vi "PostSub Steps HV PPS.vi"(0 "Sequence Context In":refnum<k7>, 1 "PPS Config In":T1={"VISA Resource"="", "Voltage Level (0.0 V)"=0.0, "CURRent Limit (0.0 A)"=0.0, "OVP LEVEL (0V)"=0.0, "Enable OVP (T: Enable)"=TRUE, "OCP LEVEL (0A)"=0.0, "Enable OCP (T: Enable)"=TRUE, "Value Out"="", "Value In"="", "Actual Voltage Level (V)"=0.0, "Actual Current Limit (A)"=0.0, "Select Instrument"="", "Enable Output"=FALSE, "PPS Operation"=enum."Close", "Type"=0} {"Type" items=["Voltage", "Current"]; "Actual Current Limit (A)" format="%.2f"; "Actual Voltage Level (V)" format="%.2f"; "OCP LEVEL (0A)" format="%.2f"; "OVP LEVEL (0V)" format="%.2f"; "Voltage Level (0.0 V)" format="%.2f"}, 2 "Socket Index":i16) -> (7 "Report Text":string, 8 "PPS Config Out":T1={"VISA Resource"="", "Voltage Level (0.0 V)"=0.0, "CURRent Limit (0.0 A)"=0.0, "OVP LEVEL (0V)"=0.0, "Enable OVP (T: Enable)"=TRUE, "OCP LEVEL (0A)"=0.0, "Enable OCP (T: Enable)"=TRUE, "Value Out"="", "Value In"="", "Actual Voltage Level (V)"=0.0, "Actual Current Limit (A)"=0.0, "Select Instrument"="", "Enable Output"=FALSE, "PPS Operation"=enum."Close", "Type"=0} {"Type" items=["Voltage", "Current"]; "Actual Current Limit (A)" format="%.2f"; "Actual Voltage Level (V)" format="%.2f"; "OCP LEVEL (0A)" format="%.2f"; "OVP LEVEL (0V)" format="%.2f"; "Voltage Level (0.0 V)" format="%.2f"}, 10 "error out":errorcluster)   [LabVIEW 2023, in "LTT_TeststandSteptypes.lvlib"]
uses:
  LTT_TeststandSteptypes.lvlib
  HardwareAbstractionLayer_LVOOP/PowerSupply/Teststand/Control/PPS StepType Control.ctl
  HardwareAbstractionLayer_LVOOP/PowerSupply/Control/PPS FGV Option.ctl
  HardwareAbstractionLayer_LVOOP/PowerSupply/Control/PPS Configure Data.ctl
  HardwareAbstractionLayer_LVOOP/PowerSupply/IT-M6018C/IT-M6018C.lvclass
  D:/eDCU LTT/VT LTT Project/Source Code/HardwareAbstractionLayer_LVOOP/PowerSupply/PowerSupply.lvclass
  <vilib>/addons/TestStand/_TSUtility.llb/TestStand - Set Property Value (Number).vi
  HardwareAbstractionLayer_LVOOP/PowerSupply/PowerSupply.lvclass
  HardwareAbstractionLayer_LVOOP/PowerSupply/IT-M3904D/IT-M3904D.lvclass
  HardwareAbstractionLayer_LVOOP/Database/Database.lvclass
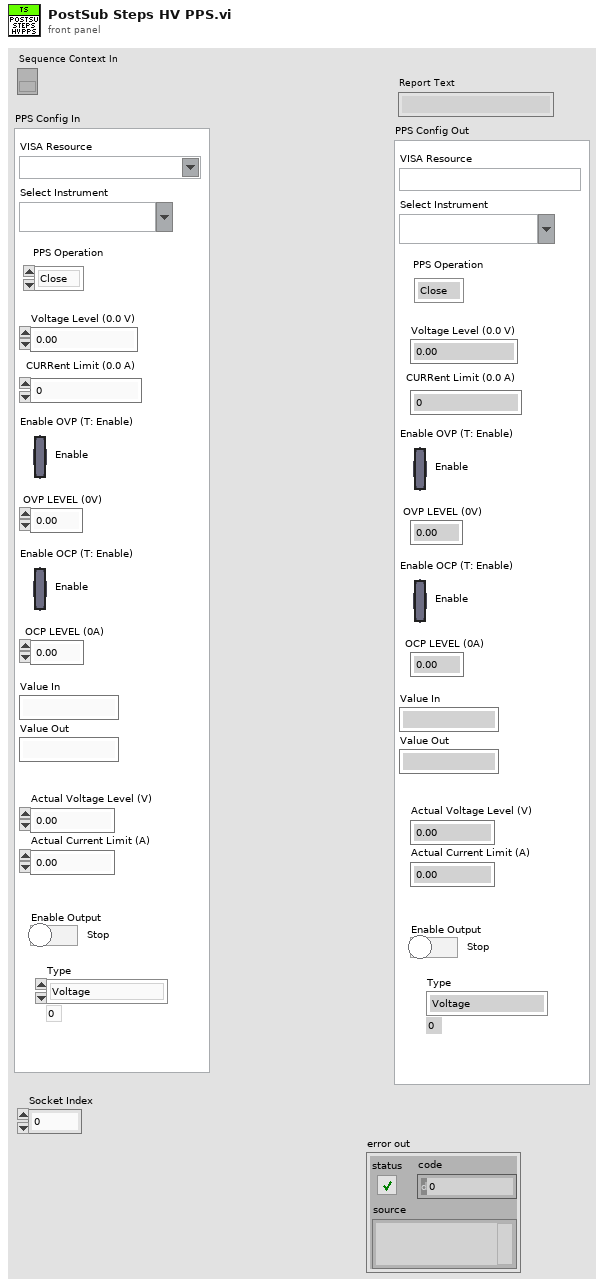
[diagram p1: front panel]
types:
  T1 = typedef "HardwareAbstractionLayer_LVOOP.lvlib/PowerSupply.lvclass/PPS StepType Control.ctl" = cluster{"VISA Resource":refnum<visa-resource-name>, "Voltage Level (0.0 V)":dbl, "CURRent Limit (0.0 A)":dbl, "OVP LEVEL (0V)":dbl, "Enable OVP (T: Enable)":bool, "OCP LEVEL (0A)":dbl, "Enable OCP (T: Enable)":bool, "Value Out":string, "Value In":string, "Actual Voltage Level (V)":dbl, "Actual Current Limit (A)":dbl, "Select Instrument":string, "Enable Output":bool, "PPS Operation":enum32{"Init", "Self Test", "Configure", "Measure", "Close"}, "Type":u16}
  T2 = enum32{"Init", "Self Test", "Configure", "Measure", "Close"}
  T3 = typedef "HardwareAbstractionLayer_LVOOP.lvlib/PowerSupply.lvclass/PPS FGV Option.ctl" = enum16{"Init Ref", "Get Ref", "Set Ref"}
  T4 = typedef "HardwareAbstractionLayer_LVOOP.lvlib/PowerSupply.lvclass/PPS Configure Data.ctl" = cluster{"Voltage Level (0.0 V)":dbl, "CURRent Limit (0.0 A)":dbl, "OVP LEVEL (0V)":dbl, "OCP LEVEL (0A)":dbl, "Enable OVP (T: Enable)":bool, "Enable OCP (T: Enable)":bool, "Enable Output ":bool, "Delays OCP":dbl, "Delays OVP":dbl, "Mode(0:Voltage)":u16, "CURRent Level (0.0 A)":dbl, "Voltage Limit (0.0 V)":dbl}
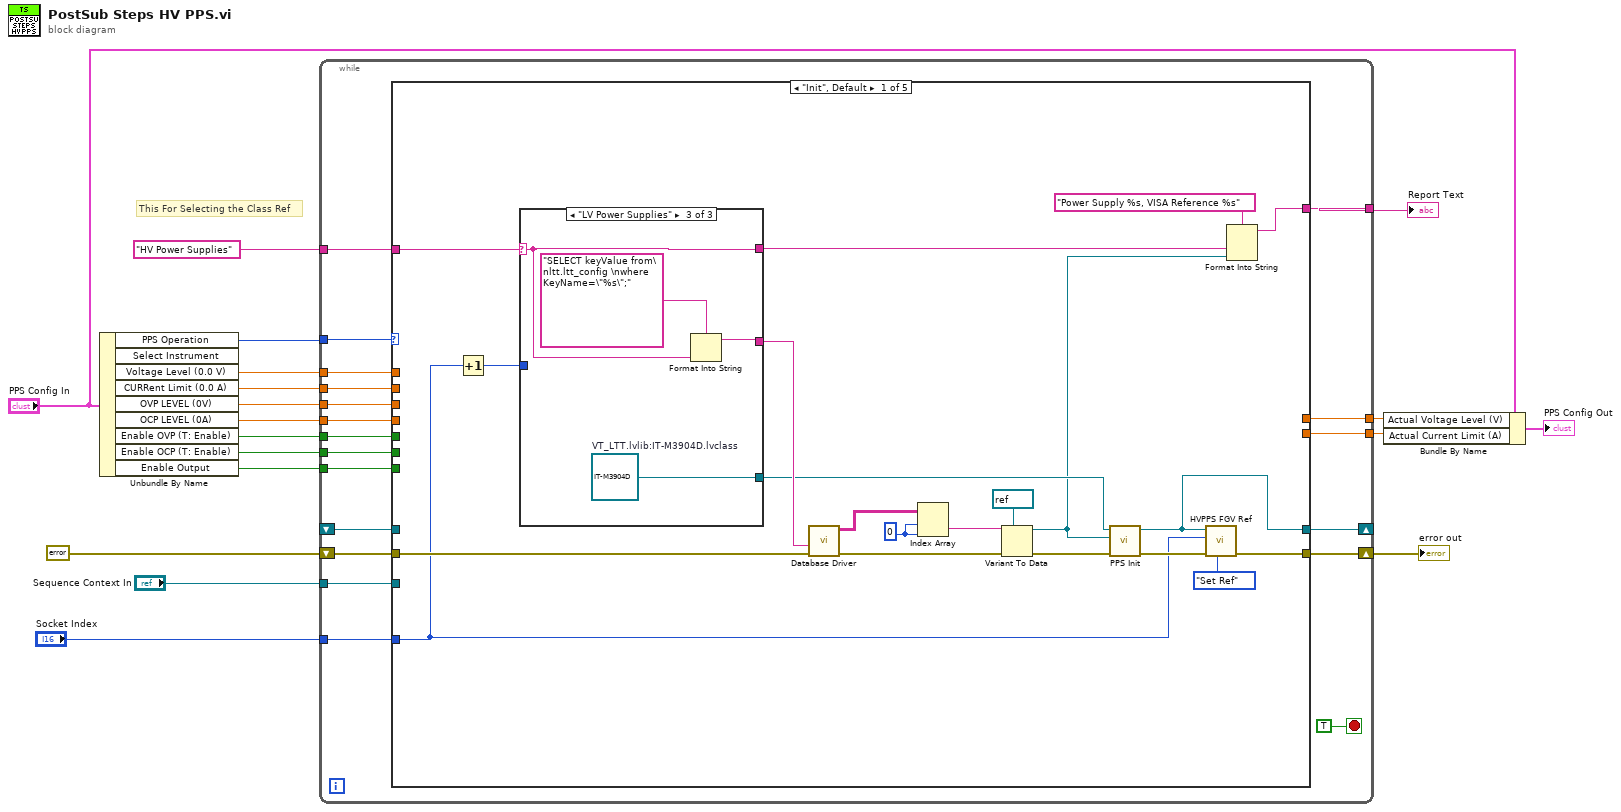
[diagram p0: block diagram]
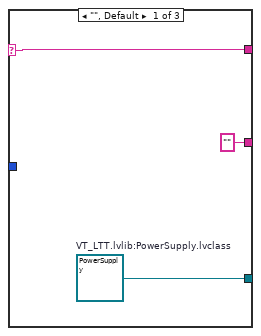
[diagram p2: hidden frame]
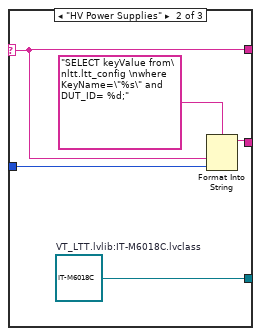
[diagram p3: hidden frame]
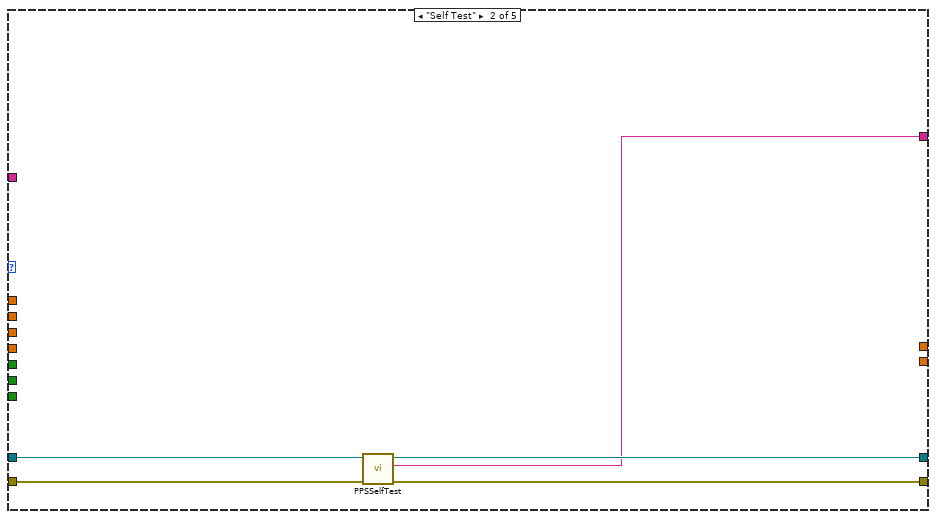
[diagram p4: hidden frame]
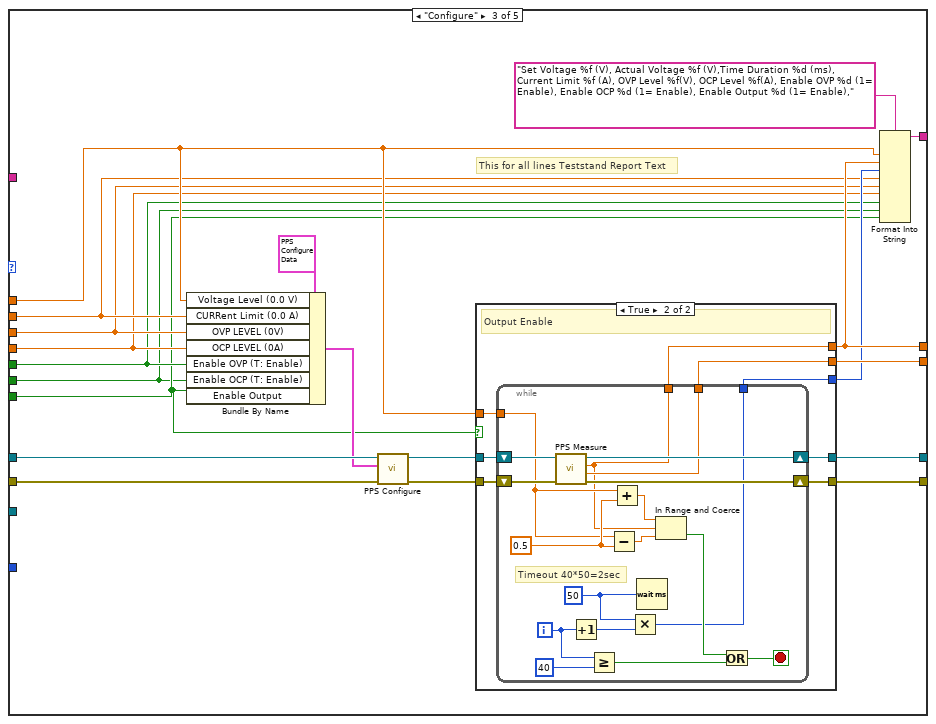
[diagram p5: hidden frame]
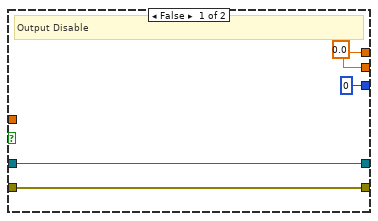
[diagram p6: hidden frame]
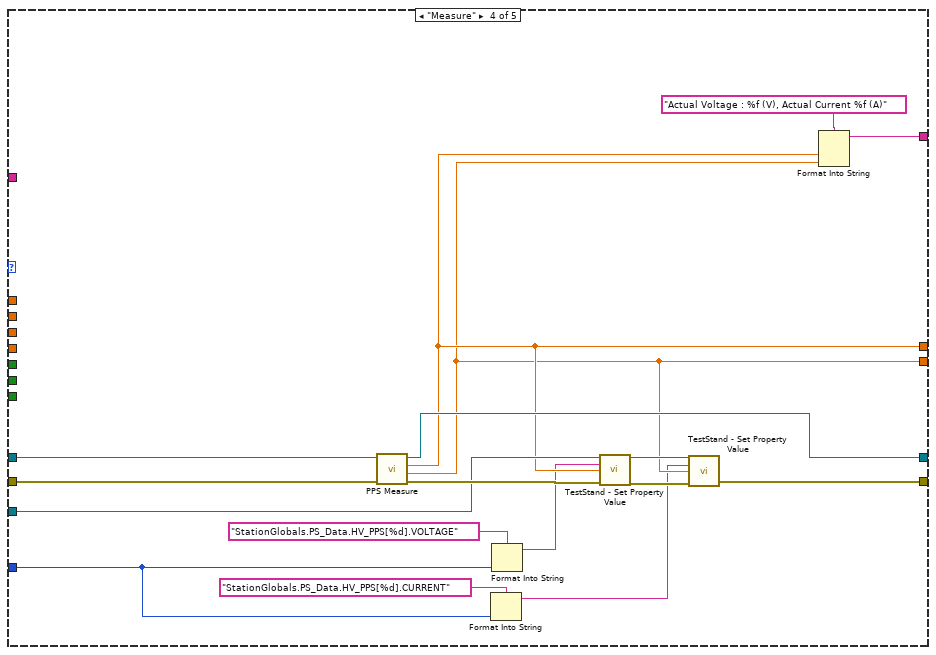
[diagram p7: hidden frame]
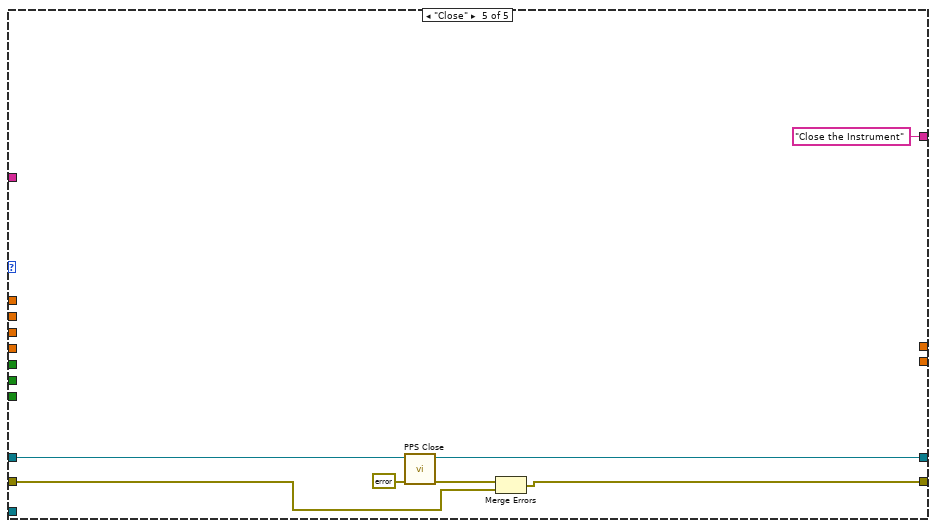
[diagram p8: hidden frame]
diagram:
  # "This For Selecting the Class Ref"
  n1 = Unbundle By Name("PPS Config In") -> ("PPS Operation"=w18:T2, "Voltage Level (0.0 V)"=w15:dbl, "CURRent Limit (0.0 A)"=w14:dbl, "OVP LEVEL (0V)"=w13:dbl, "OCP LEVEL (0A)"=w12:dbl, "Enable OVP (T: Enable)"=w11:bool, "Enable OCP (T: Enable)"=w10:bool, "Enable Output"=w9:bool)  [unwired: 1 out]
  n2 = while {
    tunnel: w18 -> [w36]
    tunnel: "HV Power Supplies" ("Select Instrument") -> [w35]
    shift-right: [w19] -> _
    shift-left: _ -> [w32]
    shift-right: [w33] -> w16
    shift-left: errorcluster {"status"=FALSE, "code"=0, "source"=""} ("error in") -> [w34]
    tunnel: w15 -> [w31]
    tunnel: w14 -> [w30]
    tunnel: w13 -> [w29]
    tunnel: w12 -> [w28]
    tunnel: w11 -> [w27]
    tunnel: w10 -> [w26]
    tunnel: w9 -> [w25]
    tunnel: [w24] -> w8
    tunnel: [w23] -> w5
    tunnel: [w22] -> w4
    tunnel: "Sequence Context In" -> [w21]
    tunnel: "Socket Index" -> [w20]
    stop <- TRUE stop-if-true
    n3 = case shown="\"Init\", Default" w36 {
      tunnel: w35 -> [w57 _ _ _ _]
      tunnel: w34 -> [w50 w73 w93 w140 w142]
      tunnel: [w41 w72 w90 w134 w143] -> w33
      tunnel: [w40 w71 w89 w139 w146] -> w19
      tunnel: w32 -> [_ w74 w94 w141 w147]
      tunnel: w31 -> [_ _ w86 _ _]
      tunnel: w30 -> [_ _ w80 _ _]
      tunnel: w29 -> [_ _ w79 _ _]
      tunnel: w28 -> [_ _ w78 _ _]
      tunnel: w27 -> [_ _ w77 _ _]
      tunnel: w26 -> [_ _ w75 _ _]
      tunnel: w25 -> [_ _ w76 _ _]
      tunnel: [w47 w70 w85 w137 "Close the Instrument" ("Self-Test Result Message")] -> w24
      tunnel: [_ _ w84 w131 _] -> w23
      tunnel: [_ _ w83 w130 _] -> w22
      tunnel: w21 -> [_ _ _ w133 _]
      tunnel: w20 -> [w39 _ _ w126 _]
      frame "Init", Default {
        w56 = 0 ("index (row)")
        n4 = Increment(x=w39) -> (x+1=w43:i16)
        n5 = case shown="\"LV Power Supplies\"" w57 {
          selector: w57 -> [w58 w62 w66]
          tunnel: [w60 w65 w69] -> w48
          tunnel: ["" w63 w67] -> w52
          tunnel: [w58 w62 w66] -> w45
          tunnel: w43 -> [_ w61 _]
          frame "", Default {
            w60 = refnum<class "PowerSupply.lvclass"> refnum  # VT_LTT.lvlib:PowerSupply.lvclass
          }
          frame "HV Power Supplies" {
            w65 = refnum<class "IT-M6018C.lvclass"> refnum  # VT_LTT.lvlib:IT-M6018C.lvclass
            n6 = Format Into String(format string="SELECT keyValue from\nltt.ltt_config \nwhere KeyName=\"%s\" and DUT_ID= %d;", w62, w61) -> (resulting string=w63:string)  [unwired: 2 in, 1 out]
          }
          frame "LV Power Supplies" {
            w69 = refnum<class "IT-M3904D.lvclass"> refnum  # VT_LTT.lvlib:IT-M3904D.lvclass
            n7 = Format Into String(format string="SELECT keyValue from\nltt.ltt_config \nwhere KeyName=\"%s\";", w66) -> (resulting string=w67:string)  [unwired: 2 in, 1 out]
          }
        }
        n8 = call "Database Driver.vi"("error in"=w50, "SQL query"=w52) -> ("error out"=w49:errorcluster, "data"=w51:string[][])  [unwired: 6 in, 2 out]
        n9 = Index Array(array=w51, index (row)=w56, index (col)=w56) -> (element=w53:string)
        n10 = Variant To Data(error in=w49, type=refnum<visa-resource-name> "LV" ("VISA resource name"), Variant=w53) -> (data=w44:refnum<visa-resource-name>, error out=w55:errorcluster)
        n11 = call-dynamic "PPS Init.vi"("error in (no error)"=w55, "VISA resource name"=w44, "PowerSupply in"=w48) -> ("error out"=w42:errorcluster, "PowerSupply out"=w40:refnum<class "PowerSupply.lvclass">)  [unwired: 7 in]
        n12 = call "HVPPS FGV Ref.vi"("Option"=PPS_FGV_Option."Set Ref", "error in"=w42, "Socket No"=w39, "PowerSupplyIn.lvclass"=w40) -> ("error out"=w41:errorcluster)  [unwired: 6 in, 1 out]
        n13 = Format Into String(format string="Power Supply %s, VISA Reference %s", w45, w44) -> (resulting string=w47:string)  [unwired: 2 in, 1 out]
      }
      frame "Self Test" {
        n14 = call-dynamic "PPSSelfTest.vi"("error in (no error)"=w73, "PowerSupply in"=w74) -> ("error out"=w72:errorcluster, "Self-Test Result Message"=w70:string, "PowerSupply out"=w71:refnum<class "PowerSupply.lvclass">)  [unwired: 7 in]
      }
      frame "Configure" {
        # "This for all lines Teststand Report Text"
        n15 = Bundle By Name(cluster=T4 {"Voltage Level (0.0 V)"=0.0, "CURRent Limit (0.0 A)"=0.0, "OVP LEVEL (0V)"=0.0, "OCP LEVEL (0A)"=0.0, "Enable OVP (T: Enable)"=TRUE, "Enable OCP (T: Enable)"=TRUE, "Enable Output "=TRUE, "Delays OCP"=0.0, "Delays OVP"=0.0, "Mode(0:Voltage)"=0, "CURRent Level (0.0 A)"=0.0, "Voltage Limit (0.0 V)"=0.0} ("Configure"), "Voltage Level (0.0 V)"=w86, "CURRent Limit (0.0 A)"=w80, "OVP LEVEL (0V)"=w79, "OCP LEVEL (0A)"=w78, "Enable OVP (T: Enable)"=w77, "Enable OCP (T: Enable)"=w75, "Enable Output"=w76) -> (w91:T4)
        n16 = call-dynamic "PPS Configure.vi"("error in (no error)"=w93, "Configure"=w91, "PowerSupply in"=w94) -> ("error out"=w82:errorcluster, "PowerSupply out"=w88:refnum<class "PowerSupply.lvclass">)  [unwired: 7 in]
        n17 = case shown="True" w76 {
          tunnel: w82 -> [w97 w106]
          tunnel: [w97 w105] -> w90
          tunnel: [w98 w104] -> w89
          tunnel: w88 -> [w98 w103]
          tunnel: w86 -> [_ w100]
          tunnel: [w96 w102] -> w84
          tunnel: [w96 w101] -> w83
          tunnel: [u32 0 w99] -> w81
          frame False {
            w96 = 0.0 ("Actual Voltage Level (V)")
            # "Output Disable"
          }
          frame True {
            # "Output Enable"
            n18 = while {
              tunnel: [w112] -> w102
              tunnel: [w120] -> w101
              shift-right: [w123] -> w105
              shift-left: w106 -> [w124]
              shift-right: [w122] -> w104
              shift-left: w103 -> [w121]
              tunnel: w100 -> [w113]
              tunnel: [w110] -> w99
              i -> [w109]
              stop <- w117 stop-if-true
              w115 = 0.5
              w111 = u32 50 ("milliseconds to wait")
              # "Timeout 40*50=2sec"
              n19 = call-dynamic "PPS Measure.vi"("error in (no error)"=w124, "PowerSupply in"=w121) -> ("error out"=w123:errorcluster, "Actual Current Limit (A)"=w120:dbl, "Actual Voltage Level (V)"=w112:dbl, "PowerSupply out"=w122:refnum<class "PowerSupply.lvclass">)  [unwired: 6 in]
              n20 = Increment(x=w109) -> (x+1=w107:i32)
              n21 = Greater Or Equal?(x=w109, y=40) -> (x >= y?=w119:bool)
              n22 = Subtract(x=w113, y=w115) -> (x-y=w114:dbl)
              n23 = Add(x=w113, y=w115) -> (x+y=w116:dbl)
              n24 = Multiply(x=w111, y=w107) -> (x*y=w110:u32)
              n25 = Wait (ms)(milliseconds to wait=w111) -> ()  [unwired: 1 out]
              n26 = In Range and Coerce(upper limit=w116, x=w112, lower limit=w114) -> (In Range?=w118:bool)  [unwired: 1 out]
              n27 = Or(x=w118, y=w119) -> (x .or. y?=w117:bool)
            }
          }
        }
        n28 = Format Into String(format string="Set Voltage %f (V), Actual Voltage %f (V),Time Duration %d (ms), Current Limit %f (A), OVP Level %f(V), OCP Level %f(A), Enable OVP %d (1= Enable), Enable OCP %d (1= Enable), Enable Output %d (1= Enable),", w86, w84, w81, w80, w79, w78, w77, w75, w76) -> (resulting string=w85:string)  [unwired: 2 in, 1 out]
      }
      frame "Measure" {
        n29 = call-dynamic "PPS Measure.vi"("error in (no error)"=w140, "PowerSupply in"=w141) -> ("error out"=w136:errorcluster, "Actual Current Limit (A)"=w130:dbl, "Actual Voltage Level (V)"=w131:dbl, "PowerSupply out"=w139:refnum<class "PowerSupply.lvclass">)  [unwired: 6 in]
        n30 = Format Into String(format string="StationGlobals.PS_Data.HV_PPS[%d].CURRENT" ("Lookup String"), w126) -> (resulting string=w125:string)  [unwired: 2 in, 1 out]
        n31 = Format Into String(format string="StationGlobals.PS_Data.HV_PPS[%d].VOLTAGE" ("Lookup String"), w126) -> (resulting string=w128:string)  [unwired: 2 in, 1 out]
        n32 = call-poly <vilib>:"TestStand - Set Property Value.vi"("Sequence Context In"=w133, "Lookup String"=w128, "New Value"=w131, "error in (no error)"=w136) -> ("Sequence Context Out"=w132:refnum<k7>, "error out"=w135:errorcluster)  [unwired: 10 in]
        n33 = call-poly <vilib>:"TestStand - Set Property Value.vi"("Sequence Context In"=w132, "Lookup String"=w125, "New Value"=w130, "error in (no error)"=w135) -> ("error out"=w134:errorcluster)  [unwired: 10 in, 1 out]
        n34 = Format Into String(format string="Actual Voltage : %f (V), Actual Current %f (A)", w131, w130) -> (resulting string=w137:string)  [unwired: 2 in, 1 out]
      }
      frame "Close" {
        n35 = call-dynamic "PPS Close.vi"("error in (no error)"=errorcluster {"status"=FALSE, "code"=0, "source"=""}, "PowerSupply in"=w147) -> ("error out"=w148:errorcluster, "PowerSupply out"=w146:refnum<class "PowerSupply.lvclass">)  [unwired: 8 in]
        n36 = Merge Errors(w148, w142) -> (w143:errorcluster)
      }
    }
  }
  "error out" <- w16
  "Report Text" <- w8
  n37 = Bundle By Name(cluster="PPS Config In", "Actual Voltage Level (V)"=w5, "Actual Current Limit (A)"=w4) -> (→"PPS Config Out":T1)
